vi "Write WebSocket Server Enqueuer.vi"(8 "error in (no error)":errorcluster, 10 "Actor Framework:Message Enqueuer":refnum<class "Message Enqueuer.lvclass">, 11 "WS Test Server in":refnum<class "WS Server.lvclass">) -> (0 "error out":errorcluster, 3 "WS Test Server out":refnum<class "WS Server.lvclass">)   [LabVIEW 2021, in "Echo Broadcast with External Client.lvlib" / "WS Server.lvclass"]
uses:
  WS Server.lvclass
  <vilib>/ActorFramework/Message Enqueuer/Message Enqueuer.lvclass
  WS Server.lvclass/WS Server.ctl
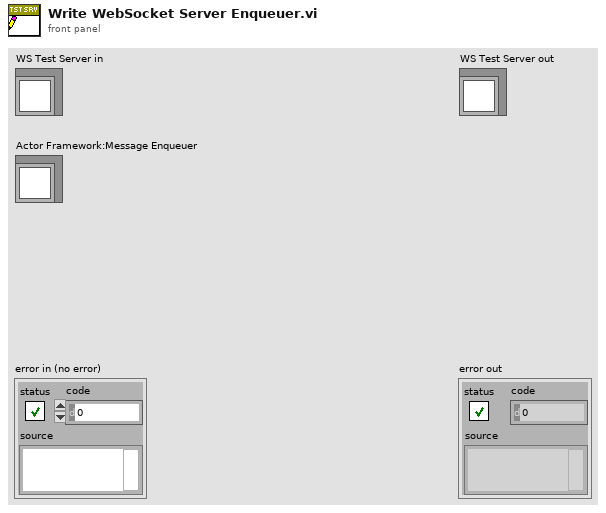
[diagram p1: front panel]
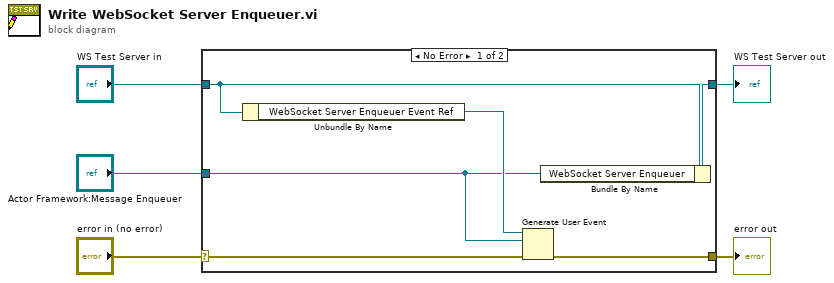
[diagram p0: block diagram]
diagram:
  n1 = case shown="No Error" "error in (no error)" {
    selector: "error in (no error)" -> [w9 w12]
    tunnel: [w8 w12] -> w4
    tunnel: [w11 w13] -> w2
    tunnel: "WS Test Server in" -> [w10 w13]
    tunnel: "Actor Framework:Message Enqueuer" -> [w6 _]
    frame No Error {
      n2 = Unbundle By Name(w10) -> ("WebSocket Server Enqueuer Event Ref"=w7:refnum<user-event>)
      n3 = Generate User Event(user event=w7, event data cluster=w6, error in=w9) -> (error out=w8:errorcluster)  [unwired: 1 in, 1 out]
      n4 = Bundle By Name(cluster=w10, "WebSocket Server Enqueuer"=w6) -> (w11:refnum<class "WS Server.lvclass">)
    }
    frame Error {
    }
  }
  "error out" <- w4
  "WS Test Server out" <- w2
